vi "Read Params from INI Section.vi"(8 "error in (no error)":errorcluster, 9 "Parameters In":variant, 10 "Refnum in":T1, 11 "Analyze BaseClass in":refnum<class "Analyze BaseClass.lvclass">) -> (0 "error out":errorcluster, 1 "Parameters Out":variant, 2 "Refnum out":T1, 3 "Analyze BaseClass out":refnum<class "Analyze BaseClass.lvclass">)   [LabVIEW 2014, in "Analyze.lvlib" / "Analyze BaseClass.lvclass"]
uses:
  Analyze BaseClass.lvclass
  <vilib>/Utility/config.llb/Config Data RefNum.ctl
  <vilib>/Utility/config.llb/NI_LVConfig.lvlib
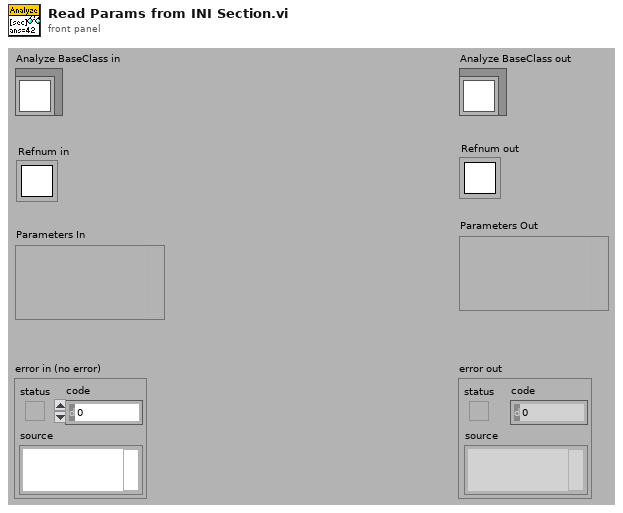
[diagram p1: front panel]
types:
  T1 = typedef "NI_LVConfig.lvlib/Config Data RefNum.ctl" = refnum<k1>
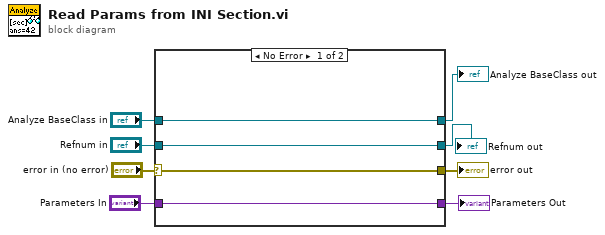
[diagram p0: block diagram]
diagram:
  n1 = case shown="No Error" "error in (no error)" {
    selector: "error in (no error)" -> [w11 w16]
    tunnel: [w11 w16] -> w7
    tunnel: [w10 w15] -> w5
    tunnel: "Analyze BaseClass in" -> [w10 w15]
    tunnel: [w12 w14] -> w4
    tunnel: "Refnum in" -> [w12 w14]
    tunnel: [w9 w13] -> w2
    tunnel: "Parameters In" -> [w9 w13]
    frame No Error {
    }
    frame Error {
    }
  }
  "error out" <- w7
  "Analyze BaseClass out" <- w5
  "Parameters Out" <- w2
  "Refnum out" <- w4
